vi "Baseline searching.vi"(4 "dt":dbl=0.0001 format="%#_13g", 6 "Matched Index":i16, 7 "배열":dbl[](array[numeric])) -> ()   [LabVIEW 2017]
uses:
  <vilib>/Analysis/NI_AALPro.lvlib
panel:
  out "최소 인덱스":i32
  out "최소값":dbl
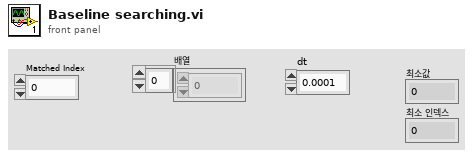
[diagram p1: front panel]
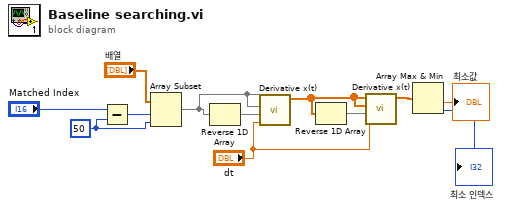
[diagram p0: block diagram]
diagram:
  w9 = i16 50 ("y")
  n1 = Subtract(x="Matched Index", y=w9) -> (x-y=w10:i16)
  n2 = Array Subset(array="배열", index=w10, length=w9) -> (w7:dbl[])
  n3 = Reverse 1D Array(array=w7) -> (reversed array=w8:dbl[])
  n4 = call <vilib>:"Derivative x(t).vi"("dt"="dt", "Final Condition"=w8, "Initial Condition"=w7, "X"=w7) -> ("dX/dt"=w5:dbl[])  [unwired: 6 in, 1 out]
  n5 = Reverse 1D Array(array=w5) -> (reversed array=w6:dbl[])
  n6 = call <vilib>:"Derivative x(t).vi"("dt"="dt", "Final Condition"=w6, "Initial Condition"=w5, "X"=w5) -> ("dX/dt"=w3:dbl[])  [unwired: 6 in, 1 out]
  n7 = Array Max & Min(array=w3) -> (min value=→"최소값":dbl, min index (indices)=→"최소 인덱스":i32)  [unwired: 2 out]
